vi "log analysis_gps.vi"() -> ()   [LabVIEW 2019] (continued)
37.37102056914,126.72168651879,7.9675,22.3000,0.3602,0.2584,-0.0273,-0.124586841,-0.381382122,33.473261992,0.4158,0.2973,0.5713,0.1134,0.0948,0.0862,0.2649,0.2392,5.1601,0f000001,0*eba26ee8\n\t", "INSPVAXA,USB3,0,50.5,FINESTEERING,2107,281412.850,02000000,471d,15824;INS_ALIGNMENT_COMPLETE,INS_RTKFIXED,37.37102404142,126.72168963423,7.9673,22.3000,0.3604,0.2695,-0.0148,-0.373966632,-0.606948860,33.415990980,0.4147,0.2955,0.5683,0.1128,0.0939,0.0847,0.2648,0.2392,5.1618,0f000001,0*2af052bc\n\t", "INSPVAXA,USB3,0,50.0,FINESTEERING,2107,281413.850,02000000,471d,15824;INS_ALIGNMENT_COMPLETE,INS_RTKFIXED,37.37102747823,126.72169275298,7.9678,22.3000,0.3771,0.2870,-0.0120,-0.268357218,-0.590747606,33.358928926,0.4139,0.2944,0.5647,0.1119,0.0930,0.0833,0.2648,0.2392,5.1630,0f000001,0*49d73869\n\t", "INSPVAXA,USB3,0,52.0,FINESTEERING,2107,281414.350,02000000,471d,15824;INS_ALIGNMENT_COMPLETE,INS_RTKFIXED,37.37102919906,126.72169428812,7.9675,22.3000,0.3604,0.2661,-0.0032,-0.659688126,-0.428969393,33.411905662,0.4132,0.2936,0.5618,0.1122,0.0937,0.0832,0.2648,0.2392,5.1641,0f000001,0*c98d060a\n\t", "INSPVAXA,USB3,0,44.5,FINESTEERING,2107,281415.350,02000000,471d,15824;INS_ALIGNMENT_COMPLETE,INS_RTKFIXED,37.37103267995,126.72169744869,7.9665,22.3000,0.3768,0.2993,-0.0116,-0.528478591,-0.759705931,33.438134045,0.4126,0.2929,0.5591,0.1118,0.0933,0.0820,0.2647,0.2392,5.1652,0f000001,0*581dc28c\n\t", "INSPVAXA,USB3,0,48.5,FINESTEERING,2107,281416.350,02000000,471d,15824;INS_ALIGNMENT_COMPLETE,INS_RTKFIXED,37.37103613052,126.72170062414,7.9635,22.3000,0.4087,0.2756,-0.0246,-0.725160800,-0.633419776,33.720037993,0.4128,0.2920,0.5564,0.1119,0.0930,0.0810,0.2647,0.2392,5.1665,0f000001,0*1631f0a5\n\t", "INSPVAXA,USB3,0,48.5,FINESTEERING,2107,281417.350,02000000,471d,15824;INS_ALIGNMENT_COMPLETE,INS_RTKFIXED,37.37103952444,126.72170377706,7.9632,22.3000,0.3570,0.2779,-0.0018,-0.570124026,-0.772949889,33.647986362,0.4118,0.2899,0.5509,0.1122,0.0932,0.0810,0.2645,0.2391,5.1675,0f000001,0*233b5573\n\t", "INSPVAXA,USB3,0,48.5,FINESTEERING,2107,281417.850,02000000,471d,15824;INS_ALIGNMENT_COMPLETE,INS_RTKFIXED,37.37104128675,126.72170534574,7.9659,22.3000,0.3708,0.2756,-0.0283,-0.789006262,-0.544112673,33.784716774,0.4118,0.2899,0.5509,0.1122,0.0932,0.0810,0.2645,0.2391,5.1675,0f000001,0*dc8c1e25\n\t", "INSPVAXA,USB3,0,49.0,FINESTEERING,2107,281418.850,02000000,471d,15824;INS_ALIGNMENT_COMPLETE,INS_RTKFIXED,37.37104464340,126.72170847296,7.9663,22.3000,0.3685,0.2500,0.0007,-0.664002073,-0.601650927,33.708955665,0.4113,0.2892,0.5478,0.1120,0.0929,0.0802,0.2644,0.2390,5.1688,0f000001,0*3627658d\n\t", "INSPVAXA,USB3,0,49.5,FINESTEERING,2107,281420.350,02000000,471d,15824;INS_ALIGNMENT_COMPLETE,INS_RTKFIXED,37.37104977182,126.72171326330,7.9681,22.3000,0.3654,0.2752,-0.0075,-0.486218413,-0.454617535,33.615388991,0.4147,0.2981,0.5609,0.1124,0.0945,0.0810,0.2643,0.2389,5.1711,0f000001,0*c1b15c55\n\t", "INSPVAXA,USB3,0,49.0,FINESTEERING,2107,281421.850,02000000,471d,15824;INS_ALIGNMENT_COMPLETE,INS_RTKFIXED,37.37105483304,126.72171804762,7.9714,22.3000,0.3720,0.2729,0.0059,-0.226869294,-0.357217167,33.322901739,0.4153,0.3006,0.5651,0.1122,0.0940,0.0806,0.2643,0.2388,5.1727,0f000001,0*c9d844c6\n\t", "INSPVAXA,USB3,0,50.0,FINESTEERING,2107,281440.400,02000000,471d,15824;INS_ALIGNMENT_COMPLETE,INS_RTKFIXED,37.37111948466,126.72177620543,7.8818,22.3000,0.3548,0.3148,0.0036,-0.259281902,-0.804731473,33.477876522,0.4069,0.2838,0.5238,0.1105,0.0914,0.0781,0.2627,0.2373,5.1917,0f000001,0*1022e28e\n\t", "INSPVAXA,USB3,0,47.0,FINESTEERING,2107,281451.400,02000000,471d,15824;INS_ALIGNMENT_COMPLETE,INS_RTKFIXED,37.37115737794,126.72181140198,7.8793,22.3000,0.3546,0.3544,0.0026,0.301499965,-0.418827265,36.616680382,0.4121,0.2951,0.5421,0.1113,0.0929,0.0791,0.2623,0.2370,5.2056,0f000001,0*452f9763\n\t", "INSPVAXA,USB3,0,44.5,FINESTEERING,2107,281452.400,02000000,471d,15824;INS_ALIGNMENT_COMPLETE,INS_RTKFIXED,37.37116058120,126.72181495507,7.8824,22.3000,0.3276,0.3265,-0.0468,0.306680390,-0.455879554,38.607757832,0.4139,0.2956,0.5455,0.1116,0.0928,0.0789,0.2623,0.2370,5.2072,0f000001,0*4613d5e8\n\t", "INSPVAXA,USB3,0,44.5,FINESTEERING,2107,281452.900,02000000,471d,15824;INS_ALIGNMENT_COMPLETE,INS_RTKFIXED,37.37116210966,126.72181674670,7.8822,22.3000,0.3215,0.3514,-0.0183,0.377751174,-0.234093113,39.308354629,0.4139,0.2956,0.5455,0.1116,0.0928,0.0789,0.2623,0.2370,5.2072,0f000001,0*f7d4e910\n\t", "INSPVAXA,USB3,0,49.0,FINESTEERING,2107,281453.400,02000000,471d,15824;INS_ALIGNMENT_COMPLETE,INS_RTKFIXED,37.37116361961,126.72181857489,7.8793,22.3000,0.3370,0.3634,-0.0294,0.431370913,-0.173130172,39.969478281,0.4147,0.2957,0.5475,0.1117,0.0928,0.0786,0.2622,0.2369,5.2083,0f000001,0*84da0b27\n\t", "INSPVAXA,USB3,0,49.0,FINESTEERING,2107,281453.900,02000000,471d,15824;INS_ALIGNMENT_COMPLETE,INS_RTKFIXED,37.37116508071,126.72182041170,7.8755,22.3000,0.3222,0.3708,0.0001,0.426257094,0.020843514,40.660737153,0.4147,0.2957,0.5475,0.1117,0.0928,0.0786,0.2622,0.2369,5.2083,0f000001,0*b9aa4650\n\t", "INSPVAXA,USB3,0,47.5,FINESTEERING,2107,281455.400,02000000,471d,15824;INS_ALIGNMENT_COMPLETE,INS_RTKFIXED,37.37116944200,126.72182606901,7.8692,22.3000,0.2987,0.3736,-0.0088,0.240749777,-0.612888046,41.923306200,0.4162,0.2974,0.5511,0.1132,0.0944,0.0792,0.2618,0.2366,5.2086,0f000001,0*c27b5d3d\n\t", "INSPVAXA,USB3,0,48.0,FINESTEERING,2107,281456.900,02000000,471d,15824;INS_ALIGNMENT_COMPLETE,INS_RTKFIXED,37.37117357948,126.72183178358,7.8608,22.3000,0.3100,0.3922,-0.0117,-0.041780079,0.015103018,42.742184550,0.4159,0.2958,0.5494,0.1140,0.0949,0.0793,0.2613,0.2363,5.2090,0f000001,0*a764cc08\n\t", "INSPVAXA,USB3,0,47.5,FINESTEERING,2107,281457.900,02008000,471d,15824;INS_ALIGNMENT_COMPLETE,INS_RTKFIXED,37.37117644696,126.72183567344,7.8614,22.3000,0.3036,0.3952,-0.0191,-0.435122492,0.297928497,42.865174724,0.4156,0.2944,0.5469,0.1149,0.0954,0.0797,0.2607,0.2357,5.2097,0f000001,0*67fee73b\n\t", "INSPVAXA,USB3,0,48.0,FINESTEERING,2107,281458.400,02008000,471d,15824;INS_ALIGNMENT_COMPLETE,INS_RTKFIXED,37.37117789762,126.72183765812,7.8605,22.3000,0.2663,0.3794,0.0055,-0.186627591,0.430628544,42.799150387,0.4156,0.2930,0.5449,0.1157,0.0959,0.0801,0.2599,0.2351,5.2111,0f000001,0*353aab58\n\t", "INSPVAXA,USB3,0,48.0,FINESTEERING,2107,281458.900,02008000,471d,15824;INS_ALIGNMENT_COMPLETE,INS_RTKFIXED,37.37117931784,126.72183956069,7.8626,22.3000,0.2674,0.3686,0.0176,-0.645699086,0.378450815,42.391957050,0.4156,0.2930,0.5449,0.1157,0.0959,0.0801,0.2599,0.2351,5.2111,0f000001,0*1d8f7f17\n\t", "INSPVAXA,USB3,0,50.5,FINESTEERING,2107,281459.900,02008000,471d,15824;INS_ALIGNMENT_COMPLETE,INS_RTKFIXED,37.37118223269,126.72184333763,7.8658,22.3000,0.2701,0.3610,0.0161,-0.453997018,0.223797272,40.778453294,0.4167,0.2944,0.5456,0.1164,0.0966,0.0809,0.2589,0.2343,5.2128,0f000001,0*32172057\n\t", "INSPVAXA,USB3,0,46.5,FINESTEERING,2107,281461.400,02008000,471d,15824;INS_ALIGNMENT_COMPLETE,INS_RTKFIXED,37.37118692248,126.72184864093,7.8697,22.3000,0.3068,0.3589,-0.0063,-0.709550175,-0.051664009,37.872013250,0.4180,0.2946,0.5458,0.1159,0.0960,0.0825,0.2566,0.2324,5.2151,0f000001,0*59364c44\n\t", "INSPVAXA,USB3,0,46.5,FINESTEERING,2107,281461.900,02008000,471d,15824;INS_ALIGNMENT_COMPLETE,INS_RTKFIXED,37.37118851997,126.72185034796,7.8716,22.3000,0.2953,0.3443,0.0004,-0.635296762,0.077766272,37.199284796,0.4180,0.2946,0.5458,0.1159,0.0960,0.0825,0.2566,0.2324,5.2151,0f000001,0*e7cf6597\n\t", "INSPVAXA,USB3,0,48.0,FINESTEERING,2107,281462.400,02008000,471d,15824;INS_ALIGNMENT_COMPLETE,INS_RTKFIXED,37.37119016469,126.72185198950,7.8718,22.3000,0.3140,0.3274,-0.0278,-0.753643784,0.303209826,36.783589938,0.4170,0.2921,0.5431,0.1150,0.0951,0.0832,0.2556,0.2316,5.2152,0f000001,0*71cc871c\n\t", "INSPVAXA,USB3,0,48.0,FINESTEERING,2107,281462.900,02008000,471d,15824;INS_ALIGNMENT_COMPLETE,INS_RTKFIXED,37.37119183431,126.72185366937,7.8730,22.3000,0.3211,0.3220,0.0114,-0.696465200,0.281664462,36.480823523,0.4170,0.2921,0.5431,0.1150,0.0951,0.0832,0.2556,0.2316,5.2152,0f000001,0*b2de4003\n\t", "INSPVAXA,USB3,0,48.5,FINESTEERING,2107,281463.400,02008000,471d,15824;INS_ALIGNMENT_COMPLETE,INS_RTKFIXED,37.37119351156,126.72185532212,7.8740,22.3000,0.2696,0.3105,-0.0010,-0.845084934,0.040994289,36.443862142,0.4171,0.2926,0.5444,0.1146,0.0951,0.0842,0.2547,0.2310,5.2149,0f000001,0*1ae650cc\n\t", "INSPVAXA,USB3,0,48.5,FINESTEERING,2107,281463.900,02008000,471d,15824;INS_ALIGNMENT_COMPLETE,INS_RTKFIXED,37.37119483302,126.72185668642,7.8760,22.3000,0.1153,0.1917,-0.0076,-0.816856486,-0.145545038,36.378444891,0.4171,0.2926,0.5444,0.1146,0.0951,0.0842,0.2547,0.2310,5.2149,0f000001,0*1c1cdd38\n\t", "INSPVAXA,USB3,0,45.5,FINESTEERING,2107,281464.400,02000000,471d,15824;INS_ALIGNMENT_COMPLETE,INS_RTKFIXED,37.37119579175,126.72185768591,7.8792,22.3000,0.1971,0.2398,0.0010,-0.742386203,-0.127943073,36.538622941,0.4195,0.2979,0.5527,0.1161,0.0973,0.0858,0.2541,0.2308,5.2143,0f000001,0*24dc1fe0\n\t", "INSPVAXA,USB3,0,45.5,FINESTEERING,2107,281464.900,02000000,471d,15824;INS_ALIGNMENT_COMPLETE,INS_RTKFIXED,37.37119672915,126.72185869204,7.8846,22.3000,0.1715,0.2230,-0.0041,-0.675547372,-0.136073790,36.631506264,0.4195,0.2979,0.5527,0.1161,0.0973,0.0858,0.2541,0.2308,5.2143,0f000001,0*e856a3ba\n\t", "INSPVAXA,USB3,0,49.0,FINESTEERING,2107,281465.400,02000000,471d,15824;INS_ALIGNMENT_COMPLETE,INS_RTKFIXED,37.37119777976,126.72185974580,7.8895,22.3000,0.1707,0.2152,-0.0021,-0.795130387,-0.134235456,36.862190913,0.4216,0.3036,0.5603,0.1136,0.0955,0.0851,0.2538,0.2307,5.2127,0f000001,0*3dceb74e\n\t", "INSPVAXA,USB3,0,49.0,FINESTEERING,2107,281465.900,02000000,471d,15824;INS_ALIGNMENT_COMPLETE,INS_RTKFIXED,37.37119882408,126.72186080871,7.8935,22.3000,0.1975,0.2377,-0.0103,-0.927101285,0.026313679,37.093891060,0.4216,0.3036,0.5603,0.1136,0.0955,0.0851,0.2538,0.2307,5.2127,0f000001,0*b32abc1e\n\t", "INSPVAXA,USB3,0,45.5,FINESTEERING,2107,281466.400,02000000,471d,15824;INS_ALIGNMENT_COMPLETE,INS_RTKFIXED,37.37119994764,126.72186191360,7.8953,22.3000,0.1896,0.2516,0.0024,-0.990040985,-0.050764765,37.290261699,0.4218,0.3053,0.5656,0.1126,0.0944,0.0842,0.2536,0.2306,5.2108,0f000001,0*ab7ec7da\n\t", "INSPVAXA,USB3,0,45.5,FINESTEERING,2107,281466.900,02000000,471d,15824;INS_ALIGNMENT_COMPLETE,INS_RTKFIXED,37.37120100149,126.72186298872,7.8973,22.3000,0.1935,0.2522,-0.0026,-0.854741520,-0.119099122,37.564308734,0.4218,0.3053,0.5656,0.1126,0.0944,0.0842,0.2536,0.2306,5.2108,0f000001,0*b7c581e3\n\t", "INSPVAXA,USB3,0,48.0,FINESTEERING,2107,281467.400,02000000,471d,15824;INS_ALIGNMENT_COMPLETE,INS_RTKFIXED,37.37120208153,126.72186408522,7.8997,22.3000,0.1778,0.2253,0.0049,-0.719912945,-0.270478243,38.035475922,0.4244,0.3113,0.5828,0.1121,0.0950,0.0843,0.2538,0.2306,5.2092,0f000001,0*8e9732d5\n\t", "INSPVAXA,USB3,0,48.0,FINESTEERING,2107,281467.900,02000000,471d,15824;INS_ALIGNMENT_COMPLETE,INS_RTKFIXED,37.37120312889,126.72186517178,7.9031,22.3000,0.2039,0.2426,0.0147,-0.720629061,-0.231870268,38.725653809,0.4244,0.3113,0.5828,0.1121,0.0950,0.0843,0.2538,0.2306,5.2092,0f000001,0*c758e7ce\n\t", "INSPVAXA,USB3,0,48.5,FINESTEERING,2107,281468.400,02000000,471d,15824;INS_ALIGNMENT_COMPLETE,INS_RTKFIXED,37.37120416086,126.72186625746,7.9066,22.3000,0.2025,0.2267,-0.0001,-0.736489084,-0.165649528,39.721937458,0.4260,0.3144,0.5975,0.1120,0.0953,0.0842,0.2539,0.2306,5.2089,0f000001,0*64b5bba4\n\t", "INSPVAXA,USB3,0,48.5,FINESTEERING,2107,281468.900,02000000,471d,15824;INS_ALIGNMENT_COMPLETE,INS_RTKFIXED,37.37120515414,126.72186733248,7.9096,22.3000,0.1860,0.2130,0.0062,-0.863833957,-0.176893088,40.861857992,0.4260,0.3144,0.5975,0.1120,0.0953,0.0842,0.2539,0.2306,5.2089,0f000001,0*48502021\n\t", "INSPVAXA,USB3,0,47.5,FINESTEERING,2107,281469.400,02000000,471d,15824;INS_ALIGNMENT_COMPLETE,INS_RTKFIXED,37.37120615783,126.72186845955,7.9127,22.3000,0.1833,0.2266,0.0157,-0.922756560,-0.128393101,41.953959499,0.4267,0.3157,0.6087,0.1119,0.0952,0.0838,0.2539,0.2306,5.2092,0f000001,0*9d6cc6cc\n\t", "INSPVAXA,USB3,0,47.5,FINESTEERING,2107,281469.900,02000000,471d,15824;INS_ALIGNMENT_COMPLETE,INS_RTKFIXED,37.37120711333,126.72186961218,7.9172,22.3000,0.1882,0.2386,0.0103,-0.812681162,-0.149481379,43.058831500,0.4267,0.3157,0.6087,0.1119,0.0952,0.0838,0.2539,0.2306,5.2092,0f000001,0*7e42c462\n\t", "INSPVAXA,USB3,0,48.0,FINESTEERING,2107,281470.400,02000000,471d,15824;INS_ALIGNMENT_COMPLETE,INS_RTKFIXED,37.37120802040,126.72187075599,7.9242,22.3000,0.1759,0.2315,0.0092,-0.712389099,-0.099720322,44.115258492,0.4228,0.3076,0.5975,0.1114,0.0938,0.0818,0.2538,0.2305,5.2102,0f000001,0*4e20fbfc\n\t", "INSPVAXA,USB3,0,48.0,FINESTEERING,2107,281470.900,02000000,471d,15824;INS_ALIGNMENT_COMPLETE,INS_RTKFIXED,37.37120891997,126.72187193685,7.9313,22.3000,0.1721,0.2325,0.0046,-0.682625247,-0.034958907,44.921832107,0.4228,0.3076,0.5975,0.1114,0.0938,0.0818,0.2538,0.2305,5.2102,0f000001,0*8a1ed08d\n\t", "INSPVAXA,USB3,0,44.5,FINESTEERING,2107,281471.400,02000000,471d,15824;INS_ALIGNMENT_COMPLETE,INS_RTKFIXED,37.37120978762,126.72187309291,7.9372,22.3000,0.1737,0.2402,0.0107,-0.896905071,0.182357572,45.734122702,0.4207,0.3039,0.5902,0.1115,0.0938,0.0806,0.2537,0.2305,5.2115,0f000001,0*f5531b04\n\t", "DUALANTENNAHEADINGA,USB3,0,44.5,FINESTEERING,2107,281471.900,02000000,d426,15824;SOL_COMPUTED,NARROW_FLOAT,-1.000000000,14.722629547,3.656694651,0.0,237.736404419,180.000000000,\"631T\",22,8,8,7,04,00,20,03*d908accb\n\t", "INSPVAXA,USB3,0,44.5,FINESTEERING,2107,281472.400,02000000,471d,15824;INS_ALIGNMENT_COMPLETE,INS_RTKFIXED,37.37121145223,126.72187546991,7.9481,22.3000,0.1558,0.2299,0.0072,-0.729574410,0.299435928,46.987178524,0.4186,0.2997,0.5808,0.1119,0.0940,0.0794,0.2536,0.2304,5.2130,0f000001,0*ceccfdc7\n\t", "DUALANTENNAHEADINGA,USB3,0,44.5,FINESTEERING,2107,281472.900,02000000,d426,15824;SOL_COMPUTED,NARROW_FLOAT,-1.000000000,19.887695313,3.310185432,0.0,262.944793701,180.000000000,\"631T\",19,8,8,7,04,00,20,03*e2f42a0a\n\t", "INSPVAXA,USB3,0,47.0,FINESTEERING,2107,281473.400,02000000,471d,15824;INS_ALIGNMENT_COMPLETE,INS_RTKFIXED,37.37121309194,126.72187787297,7.9563,22.3000,0.1608,0.2402,-0.0008,-0.731141510,0.324719411,47.702294704,0.4170,0.2975,0.5726,0.1126,0.0945,0.0786,0.2534,0.2303,5.2142,0f000001,0*03d357e2\n\t", "INSPVAXA,USB3,0,47.0,FINESTEERING,2107,281473.900,02000000,471d,15824;INS_ALIGNMENT_COMPLETE,INS_RTKFIXED,37.37121388735,126.72187905524,7.9593,22.3000,0.1511,0.2341,0.0050,-0.781655169,0.200652129,47.998434662,0.4170,0.2975,0.5726,0.1126,0.0945,0.0786,0.2534,0.2303,5.2142,0f000001,0*3307b87f\n\t", "INSPVAXA,USB3,0,50.0,FINESTEERING,2107,281474.400,02000000,471d,15824;INS_ALIGNMENT_COMPLETE,INS_RTKFIXED,37.37121466825,126.72188022113,7.9625,22.3000,0.1592,0.2409,0.0043,-0.925136185,0.519912466,48.197361455,0.4159,0.2959,0.5651,0.1133,0.0951,0.0780,0.2531,0.2301,5.2153,0f000001,0*acbf0539\n\t", "DUALANTENNAHEADINGA,USB3,0,50.0,FINESTEERING,2107,281474.900,02000000,d426,15824;SOL_COMPUTED,L1_FLOAT,-1.000000000,29.703872681,-19.285949707,0.0,227.925506592,180.000000000,\"631T\",19,7,7,7,04,00,20,02*438e8014\n\t", "INSPVAXA,USB3,0,48.0,FINESTEERING,2107,281475.400,02000000,471d,15824;INS_ALIGNMENT_COMPLETE,INS_RTKFIXED,37.37121622258,126.72188269700,7.9646,22.3000,0.1441,0.2253,0.0054,-0.653688748,0.578968322,48.454145381,0.4152,0.2943,0.5583,0.1140,0.0955,0.0776,0.2526,0.2297,5.2166,0f000001,0*7e585380\n\t", "INSPVAXA,USB3,0,48.0,FINESTEERING,2107,281475.900,02000000,471d,15824;INS_ALIGNMENT_COMPLETE,INS_RTKFIXED,37.37121692154,126.72188386600,7.9655,22.3000,0.1584,0.2123,0.0124,-0.619737810,0.551987551,48.617638369,0.4152,0.2943,0.5583,0.1140,0.0955,0.0776,0.2526,0.2297,5.2166,0f000001,0*cdba2d64\n\t", "INSPVAXA,USB3,0,46.5,FINESTEERING,2107,281476.400,02000000,471d,15824;INS_ALIGNMENT_COMPLETE,INS_RTKFIXED,37.37121768155,126.72188507525,7.9668,22.3000,0.1354,0.2014,0.0180,-0.822035432,0.378941407,48.791141972,0.4147,0.2931,0.5519,0.1146,0.0957,0.0772,0.2519,0.2292,5.2180,0f000001,0*1e1562b5\n\t", "INSPVAXA,USB3,0,46.5,FINESTEERING,2107,281476.900,02000000,471d,15824;INS_ALIGNMENT_COMPLETE,INS_RTKFIXED,37.37121850161,126.72188636358,7.9688,22.3000,0.1738,0.2367,0.0108,-1.201696541,-0.232647671,48.968391321,0.4147,0.2931,0.5519,0.1146,0.0957,0.0772,0.2519,0.2292,5.2180,0f000001,0*afd5e89e\n\t", "INSPVAXA,USB3,0,50.5,FINESTEERING,2107,281477.400,02000000,471d,15824;INS_ALIGNMENT_COMPLETE,INS_RTKFIXED,37.37121929078,126.72188763502,7.9707,22.3000,0.1401,0.2321,0.0104,-1.230903565,-0.339648847,49.051409136,0.4145,0.2921,0.5464,0.1152,0.0963,0.0770,0.2510,0.2285,5.2193,0f000001,0*fd6eca37\n\t", "DUALANTENNAHEADINGA,USB3,0,50.5,FINESTEERING,2107,281477.900,02000000,d426,15824;SOL_COMPUTED,NARROW_FLOAT,-1.000000000,24.973518372,-6.230041504,0.0,279.644378662,180.000000000,\"631T\",18,8,8,6,04,00,20,03*2ec7f676\n\t", "DUALANTENNAHEADINGA,USB3,0,45.5,FINESTEERING,2107,281478.400,02000000,d426,15824;SOL_COMPUTED,NARROW_FLOAT,-1.000000000,25.984382629,-14.421966553,0.0,321.839630127,180.000000000,\"631T\",19,7,7,6,04,00,20,03*c537a035\n\t", "INSPVAXA,USB3,0,45.5,FINESTEERING,2107,281478.900,02000000,471d,15824;INS_ALIGNMENT_COMPLETE,INS_RTKFIXED,37.37122160716,126.72189152509,7.9681,22.3000,0.1537,0.2575,-0.0106,-0.771104700,-0.770425381,49.241520291,0.4142,0.2902,0.5416,0.1154,0.0959,0.0768,0.2499,0.2277,5.2192,0f000001,0*21e6a269\n\t", "INSPVAXA,USB3,0,48.0,FINESTEERING,2107,281479.400,02000000,471d,15824;INS_ALIGNMENT_COMPLETE,INS_RTKFIXED,37.37122237259,126.72189283393,7.9651,22.3000,0.1293,0.2257,0.0059,-0.612587772,-1.097823401,49.383599810,0.4139,0.2890,0.5376,0.1159,0.0956,0.0767,0.2487,0.2267,5.2174,0f000001,0*f7632e7f\n\t", "INSPVAXA,USB3,0,48.0,FINESTEERING,2107,281479.900,02000000,471d,15824;INS_ALIGNMENT_COMPLETE,INS_RTKFIXED,37.37122311792,126.72189412346,7.9647,22.3000,0.1494,0.2660,0.0073,-0.587954124,-1.340332352,49.363469621,0.4139,0.2890,0.5376,0.1159,0.0956,0.0767,0.2487,0.2267,5.2174,0f000001,0*4724fb20\n\t", "DUALANTENNAHEADINGA,USB3,0,48.5,FINESTEERING,2107,281480.400,02000000,d426,15824;SOL_COMPUTED,L1_FLOAT,-1.000000000,38.387950897,-13.434600830,0.0,360.000000000,180.000000000,\"631T\",19,7,7,7,04,00,20,02*88d00c71\n\t", "DUALANTENNAHEADINGA,USB3,0,48.5,FINESTEERING,2107,281480.900,02000000,d426,15824;SOL_COMPUTED,L1_FLOAT,-1.000000000,37.718753815,-13.467346191,0.0,360.000000000,180.000000000,\"631T\",19,7,7,7,04,00,20,02*9128bd3b\n\t", "DUALANTENNAHEADINGA,USB3,0,46.5,FINESTEERING,2107,281481.400,02008000,d426,15824;SOL_COMPUTED,NARROW_FLOAT,-1.000000000,32.154727936,-10.026550293,0.0,255.698348999,180.000000000,\"631T\",21,8,8,7,04,00,20,03*90654ace\n\t", "INSPVAXA,USB3,0,46.5,FINESTEERING,2107,281481.900,02008000,471d,15824;INS_ALIGNMENT_COMPLETE,INS_RTKFIXED,37.37122611752,126.72189916270,7.9537,22.3000,0.1376,0.2362,0.0025,-0.095529965,-0.586716272,48.576302995,0.4131,0.2860,0.5308,0.1150,0.0939,0.0764,0.2461,0.2246,5.2038,0f000001,0*d4dc6a04\n\t", "INSPVAXA,USB3,0,43.0,FINESTEERING,2107,281482.400,02008000,471d,15824;INS_ALIGNMENT_COMPLETE,INS_RTKFIXED,37.37122693129,126.72190044241,7.9507,22.3000,0.1400,0.2344,0.0009,-0.286718935,-0.542573010,48.417760410,0.4129,0.2856,0.5284,0.1143,0.0930,0.0764,0.2448,0.2237,5.1963,0f000001,0*4b0c873a\n\t", "DUALANTENNAHEADINGA,USB3,0,43.0,FINESTEERING,2107,281482.900,02008000,d426,15824;SOL_COMPUTED,NARROW_FLOAT,-1.000000000,25.759243011,-24.488281250,0.0,296.027648926,180.000000000,\"631T\",21,7,7,7,04,00,20,03*7949ae50\n\t", "DUALANTENNAHEADINGA,USB3,0,49.0,FINESTEERING,2107,281483.400,02008000,d426,15824;SOL_COMPUTED,NARROW_FLOAT,-1.000000000,21.557176590,-28.431182861,0.0,309.766693115,180.000000000,\"631T\",20,8,8,7,04,00,20,03*24e13096\n\t", "INSPVAXA,USB3,0,49.0,FINESTEERING,2107,281483.900,02008000,471d,15824;INS_ALIGNMENT_COMPLETE,INS_RTKFIXED,37.37122933882,126.72190424641,7.9440,22.3000,0.1298,0.2079,0.0016,-0.555050997,-0.344115137,48.037628133,0.4121,0.2847,0.5256,0.1130,0.0922,0.0763,0.2437,0.2229,5.1908,0f000001,0*4fcd94af\n\t", "DUALANTENNAHEADINGA,USB3,0,50.0,FINESTEERING,2107,281484.400,02008000,d426,15824;SOL_COMPUTED,L1_FLOAT,-1.000000000,37.365016937,-21.970794678,0.0,360.000000000,180.000000000,\"631T\",19,7,7,7,04,00,20,02*e133e505\n\t", "INSPVAXA,USB3,0,50.0,FINESTEERING,2107,281484.900,02008000,471d,15824;INS_ALIGNMENT_COMPLETE,INS_RTKFIXED,37.37123096597,126.72190680248,7.9384,22.3000,0.1511,0.2333,-0.0078,-0.410489938,-0.523354884,48.112153719,0.4115,0.2844,0.5237,0.1121,0.0916,0.0762,0.2426,0.2223,5.1884,0f000001,0*a1f40ef1\n\t", "DUALANTENNAHEADINGA,USB3,0,47.5,FINESTEERING,2107,281485.400,02000000,d426,15824;SOL_COMPUTED,NARROW_FLOAT,-1.000000000,34.474456787,-26.341827393,0.0,271.964752197,180.000000000,\"631T\",20,7,7,7,04,00,20,03*cc121194\n\t", "INSPVAXA,USB3,0,47.5,FINESTEERING,2107,281485.900,02000000,471d,15824;INS_ALIGNMENT_COMPLETE,INS_RTKFIXED,37.37123256957,126.72190927922,7.9317,22.3000,0.1299,0.2173,-0.0089,-0.426845608,-0.944074849,48.432879849,0.4110,0.2838,0.5218,0.1115,0.0911,0.0761,0.2417,0.2218,5.1881,0f000001,0*ee8ace9e\n\t", "DUALANTENNAHEADINGA,USB3,0,48.0,FINESTEERING,2107,281486.400,02000000,d426,15824;SOL_COMPUTED,L1_FLOAT,-1.000000000,34.864692688,-21.694915771,0.0,360.000000000,180.000000000,\"631T\",20,7,7,7,04,00,20,02*de044530\n\t", "DUALANTENNAHEADINGA,USB3,0,48.0,FINESTEERING,2107,281486.900,02000000,d426,15824;SOL_COMPUTED,L1_FLOAT,-1.000000000,35.417118073,-21.326538086,0.0,360.000000000,180.000000000,\"631T\",20,7,7,7,04,00,20,02*a4d3627b\n\t", "INSPVAXA,USB3,0,48.5,FINESTEERING,2107,281487.400,02000000,471d,15824;INS_ALIGNMENT_COMPLETE,INS_RTKFIXED,37.37123510484,126.72191313192,7.9239,22.3000,0.1508,0.2267,-0.0041,-0.710611469,-0.697297129,49.092383754,0.4097,0.2833,0.5200,0.1105,0.0907,0.0760,0.2404,0.2213,5.1897,0f000001,0*65fc2fbf\n\t", "INSPVAXA,USB3,0,48.5,FINESTEERING,2107,281487.900,02000000,471d,15824;INS_ALIGNMENT_COMPLETE,INS_RTKFIXED,37.37123588578,126.72191437981,7.9197,22.3000,0.1455,0.2377,-0.0129,-0.683157100,-0.548580830,49.602033608,0.4097,0.2833,0.5200,0.1105,0.0907,0.0760,0.2404,0.2213,5.1897,0f000001,0*fc400f11\n\t", "INSPVAXA,USB3,0,47.5,FINESTEERING,2107,281488.400,02000000,471d,15824;INS_ALIGNMENT_COMPLETE,INS_RTKFIXED,37.37123668548,126.72191567046,7.9173,22.3000,0.1286,0.2563,0.0010,-0.700638856,-0.301855154,50.490709534,0.4091,0.2828,0.5195,0.1103,0.0906,0.0760,0.2400,0.2212,5.1909,0f000001,0*20940426\n\t", "INSPVAXA,USB3,0,47.5,FINESTEERING,2107,281488.900,02000000,471d,15824;INS_ALIGNMENT_COMPLETE,INS_RTKFIXED,37.37123745255,126.72191698522,7.9152,22.3000,0.1363,0.2513,-0.0110,-0.588840465,-0.298661481,51.824057860,0.4091,0.2828,0.5195,0.1103,0.0906,0.0760,0.2400,0.2212,5.1909,0f000001,0*3253a0a6\n\t", "DUALANTENNAHEADINGA,USB3,0,48.5,FINESTEERING,2107,281489.400,02000000,d426,15824;SOL_COMPUTED,NARROW_FLOAT,-1.000000000,34.332912445,-16.076080322,0.0,273.294891357,180.000000000,\"631T\",21,7,7,7,04,00,20,02*2e8f18b8\n\t", "DUALANTENNAHEADINGA,USB3,0,48.5,FINESTEERING,2107,281489.900,02000000,d426,15824;SOL_COMPUTED,NARROW_FLOAT,-1.000000000,35.701751709,-15.985229492,0.0,272.194824219,180.000000000,\"631T\",19,7,7,7,04,00,20,03*54912f65\n\t", "DUALANTENNAHEADINGA,USB3,0,49.0,FINESTEERING,2107,281490.400,02000000,d426,15824;SOL_COMPUTED,L1_FLOAT,-1.000000000,33.157665253,-11.030181885,0.0,245.857955933,180.000000000,\"631T\",19,7,7,7,04,00,20,02*0068c7a6\n\t", "INSPVAXA,USB3,0,49.0,FINESTEERING,2107,281490.900,02000000,471d,15824;INS_ALIGNMENT_COMPLETE,INS_RTKFIXED,37.37124025850,126.72192244807,7.9063,22.3000,0.0958,0.2597,0.0085,-0.741191829,-0.240876601,58.109405467,0.4082,0.2817,0.5177,0.1106,0.0906,0.0758,0.2393,0.2210,5.1939,0f000001,0*b3d0469a\n\t", "INSPVAXA,USB3,0,49.0,FINESTEERING,2107,281491.400,02000000,471d,15824;INS_ALIGNMENT_COMPLETE,INS_RTKFIXED,37.37124087093,126.72192387521,7.9056,22.3000,0.0957,0.2456,-0.0018,-0.666118734,-0.163871029,59.496681270,0.4086,0.2815,0.5172,0.1112,0.0911,0.0758,0.2390,0.2209,5.1955,0f000001,0*877ace1f\n\t", "DUALANTENNAHEADINGA,USB3,0,49.0,FINESTEERING,2107,281491.900,02000000,d426,15824;SOL_COMPUTED,L1_FLOAT,-1.000000000,38.072498322,-12.872985840,0.0,241.422912598,180.000000000,\"631T\",19,9,9,9,04,00,20,22*0432346e\n\t", "DUALANTENNAHEADINGA,USB3,0,48.5,FINESTEERING,2107,281492.400,02000000,d426,15824;SOL_COMPUTED,L1_FLOAT,-1.000000000,43.679172516,-11.013610840,0.0,278.657897949,180.000000000,\"631T\",19,9,9,9,04,00,20,22*bdfbef21\n\t", "DUALANTENNAHEADINGA,USB3,0,48.5,FINESTEERING,2107,281492.900,02000000,d426,15824;SOL_COMPUTED,L1_FLOAT,-1.000000000,44.166721344,-11.721832275,0.0,281.896148682,180.000000000,\"631T\",20,9,9,9,04,00,20,22*48a6c000\n\t", "INSPVAXA,USB3,0,42.5,FINESTEERING,2107,281493.400,02000000,471d,15824;INS_ALIGNMENT_COMPLETE,INS_RTKFIXED,37.37124296430,126.72192966667,7.9049,22.3000,0.0753,0.2701,-0.0078,-0.323936505,-0.201612973,63.426537614,0.4097,0.2821,0.5162,0.1137,0.0933,0.0757,0.2379,0.2204,5.1978,0f000001,0*1142f323\n\t", "INSPVAXA,USB3,0,42.5,FINESTEERING,2107,281493.900,02000000,471d,15824;INS_ALIGNMENT_COMPLETE,INS_RTKFIXED,37.37124340358,126.72193109595,7.9039,22.3000,0.0669,0.2621,-0.0103,-0.274820593,-0.183280206,64.003294915,0.4097,0.2821,0.5162,0.1137,0.0933,0.0757,0.2379,0.2204,5.1978,0f000001,0*917919f7\n\t", "DUALANTENNAHEADINGA,USB3,0,47.0,FINESTEERING,2107,281494.400,02000000,d426,15824;SOL_COMPUTED,L1_FLOAT,-1.000000000,39.924659729,-8.854888916,0.0,360.000000000,180.000000000,\"631T\",19,7,7,7,04,00,20,02*f82ff11c\n\t", "DUALANTENNAHEADINGA,USB3,0,47.0,FINESTEERING,2107,281494.900,02000000,d426,15824;SOL_COMPUTED,L1_FLOAT,-1.000000000,40.630737305,-7.196624756,0.0,360.000000000,180.000000000,\"631T\",19,7,7,7,04,00,20,02*f7322ed7\n\t", "DUALANTENNAHEADINGA,USB3,0,52.0,FINESTEERING,2107,281495.400,02000000,d426,15824;SOL_COMPUTED,L1_FLOAT,-1.000000000,40.645214081,-8.830108643,0.0,360.000000000,180.000000000,\"631T\",18,7,7,7,04,00,20,02*8609447b\n\t", "INSPVAXA,USB3,0,52.0,FINESTEERING,2107,281495.900,02000000,471d,15824;INS_ALIGNMENT_COMPLETE,INS_RTKFIXED,37.37124512541,126.72193695200,7.9047,22.3000,0.0463,0.2469,-0.0072,0.000083390,-0.348047959,65.534193450,0.4125,0.2835,0.5158,0.1165,0.0957,0.0756,0.2356,0.2190,5.1978,0f000001,0*14e6bfac\n\t", "DUALANTENNAHEADINGA,USB3,0,49.0,FINESTEERING,2107,281496.400,02000000,d426,15824;SOL_COMPUTED,NARROW_FLOAT,-1.000000000,36.124023438,-7.202545166,0.0,327.448486328,180.000000000,\"631T\",21,7,7,7,04,00,20,03*2df9ffe6\n\t", "DUALANTENNAHEADINGA,USB3,0,49.0,FINESTEERING,2107,281496.900,02000000,d426,15824;SOL_COMPUTED,NARROW_FLOAT,-1.000000000,36.800415039,-8.357086182,0.0,335.148284912,180.000000000,\"631T\",21,7,7,7,04,00,20,03*89694ba0\n\t", "DUALANTENNAHEADINGA,USB3,0,45.5,FINESTEERING,2107,281497.400,02000000,d426,15824;SOL_COMPUTED,NARROW_FLOAT,-1.000000000,35.379425049,-14.173278809,0.0,252.907455444,180.000000000,\"631T\",20,8,8,7,04,00,20,03*7b0cb3e2\n\t", "DUALANTENNAHEADINGA,USB3,0,45.5,FINESTEERING,2107,281497.900,02000000,d426,15824;SOL_COMPUTED,NARROW_FLOAT,-1.000000000,35.681621552,-15.419891357,0.0,255.079315186,180.000000000,\"631T\",18,8,8,7,04,00,20,03*3e48e9bf\n\t", "DUALANTENNAHEADINGA,USB3,0,47.0,FINESTEERING,2107,281498.400,02008000,d426,15824;SOL_COMPUTED,L1_FLOAT,-1.000000000,40.500751495,-12.284759521,0.0,360.000000000,180.000000000,\"631T\",19,7,7,7,04,00,20,02*8d7c2d6f\n\t", "DUALANTENNAHEADINGA,USB3,0,46.5,FINESTEERING,2107,281499.400,02008000,d426,15824;SOL_COMPUTED,L1_FLOAT,-1.000000000,47.084907532,-15.694274902,0.0,360.000000000,180.000000000,\"631T\",19,7,7,7,04,00,20,02*f0de5a60\n\t", "DUALANTENNAHEADINGA,USB3,0,46.5,FINESTEERING,2107,281499.900,02008000,d426,15824;SOL_COMPUTED,L1_FLOAT,-1.000000000,46.870197296,-16.724273682,0.0,360.000000000,180.000000000,\"631T\",18,7,7,7,04,00,20,02*32f34491\n\t", "DUALANTENNAHEADINGA,USB3,0,48.5,FINESTEERING,2107,281500.400,02008000,d426,15824;SOL_COMPUTED,L1_FLOAT,-1.000000000,46.407375336,-16.426940918,0.0,360.000000000,180.000000000,\"631T\",18,7,7,7,04,00,20,02*243e6382\n\t", "DUALANTENNAHEADINGA,USB3,0,48.5,FINESTEERING,2107,281500.900,02008000,d426,15824;SOL_COMPUTED,L1_FLOAT,-1.000000000,46.192268372,-15.498413086,0.0,360.000000000,180.000000000,\"631T\",17,7,7,7,04,00,20,02*d63e23bb\n\t", "DUALANTENNAHEADINGA,USB3,0,48.5,FINESTEERING,2107,281501.400,02008000,d426,15824;SOL_COMPUTED,L1_FLOAT,-1.000000000,48.142848969,-21.188415527,0.0,360.000000000,180.000000000,\"631T\",17,7,7,7,04,00,20,02*7f9c1701\n\t", "DUALANTENNAHEADINGA,USB3,0,48.5,FINESTEERING,2107,281501.900,02008000,d426,15824;SOL_COMPUTED,L1_FLOAT,-1.000000000,48.243919373,-21.323577881,0.0,360.000000000,180.000000000,\"631T\",18,7,7,7,04,00,20,02*9b797559\n\t", "DUALANTENNAHEADINGA,USB3,0,51.0,FINESTEERING,2107,281502.400,02000000,d426,15824;SOL_COMPUTED,L1_FLOAT,-1.000000000,54.417652130,-31.199645996,0.0,360.000000000,180.000000000,\"631T\",17,7,7,7,04,00,20,02*139cf8a7\n\t", "DUALANTENNAHEADINGA,USB3,0,51.0,FINESTEERING,2107,281504.900,02000000,d426,15824;SOL_COMPUTED,NARROW_FLOAT,-1.000000000,45.458030701,-24.170471191,0.0,349.614562988,180.000000000,\"631T\",18,7,7,7,04,00,20,03*3763f111\n\t", "DUALANTENNAHEADINGA,USB3,0,47.0,FINESTEERING,2107,281506.400,02000000,d426,15824;SOL_COMPUTED,L1_FLOAT,-1.000000000,47.490772247,-15.120605469,0.0,360.000000000,180.000000000,\"631T\",20,7,7,7,04,00,20,02*6c842724\n\t", "DUALANTENNAHEADINGA,USB3,0,47.0,FINESTEERING,2107,281506.900,02000000,d426,15824;SOL_COMPUTED,L1_FLOAT,-1.000000000,47.711154938,-15.635345459,0.0,360.000000000,180.000000000,\"631T\",18,7,7,7,04,00,20,02*a44c5d4d\n\t", "DUALANTENNAHEADINGA,USB3,0,47.5,FINESTEERING,2107,281507.400,02000000,d426,15824;SOL_COMPUTED,NARROW_FLOAT,-1.000000000,42.099899292,-18.667358398,0.0,341.481109619,180.000000000,\"631T\",17,7,7,7,04,00,20,03*b5db1bef\n\t", "INSPVAXA,USB3,0,47.5,FINESTEERING,2107,281507.950,02000000,471d,15824;INS_ALIGNMENT_COMPLETE,INS_RTKFIXED,37.37125380804,126.72197426812,7.8769,22.3000,-0.0203,0.2606,-0.0150,0.201245645,-0.677592145,78.627863448,0.4158,0.2828,0.5148,0.1162,0.0939,0.0753,0.2087,0.2003,5.2095,0f000001,0*4e226b57\n\t", "DUALANTENNAHEADINGA,USB3,0,49.0,FINESTEERING,2107,281508.900,02000000,d426,15824;SOL_COMPUTED,L1_FLOAT,-1.000000000,44.870548248,-15.658569336,0.0,360.000000000,180.000000000,\"631T\",16,7,7,7,04,00,20,02*b0c8f4ea\n\t", "DUALANTENNAHEADINGA,USB3,0,48.0,FINESTEERING,2107,281509.400,02000000,d426,15824;SOL_COMPUTED,NARROW_FLOAT,-1.000000000,43.414321899,-11.001037598,0.0,331.000732422,180.000000000,\"631T\",16,7,7,7,04,00,20,03*47deaf74\n\t", "INSPVAXA,USB3,0,48.0,FINESTEERING,2107,281509.950,02000000,471d,15824;INS_ALIGNMENT_COMPLETE,INS_RTKFIXED,37.37125445097,126.72198074425,7.8673,22.3000,-0.0085,0.2660,-0.0026,-0.121772207,-0.607137029,81.065804036,0.4154,0.2822,0.5141,0.1167,0.0945,0.0753,0.2051,0.1982,5.2122,0f000001,0*3f1eba48\n\t", "INSPVAXA,USB3,0,49.0,FINESTEERING,2107,281510.950,02000000,471d,15824;INS_ALIGNMENT_COMPLETE,INS_RTKFIXED,37.37125469386,126.72198394017,7.8637,22.3000,-0.0196,0.2391,0.0072,0.076200497,-0.660108168,81.872681824,0.4156,0.2817,0.5136,0.1168,0.0948,0.0753,0.2032,0.1971,5.2137,0f000001,0*0481949b\n\t", "DUALANTENNAHEADINGA,USB3,0,46.5,FINESTEERING,2107,281511.400,02000000,d426,15824;SOL_COMPUTED,L1_FLOAT,-1.000000000,48.665706635,-11.851898193,0.0,360.000000000,180.000000000,\"631T\",23,7,7,7,04,00,20,02*002e390f\n\t", "DUALANTENNAHEADINGA,USB3,0,46.5,FINESTEERING,2107,281511.900,02000000,d426,15824;SOL_COMPUTED,L1_FLOAT,-1.000000000,49.675540924,-13.921539307,0.0,360.000000000,180.000000000,\"631T\",22,7,7,7,04,00,20,02*d8f1bbd6\n\t", "DUALANTENNAHEADINGA,USB3,0,49.5,FINESTEERING,2107,281513.900,02000000,d426,15824;SOL_COMPUTED,NARROW_FLOAT,-1.000000000,44.284626007,-19.218811035,0.0,360.000000000,180.000000000,\"631T\",20,7,7,7,04,00,20,02*521f05df\n\t", "INSPVAXA,USB3,0,49.5,FINESTEERING,2107,281514.450,02000000,471d,15824;INS_ALIGNMENT_COMPLETE,INS_RTKFIXED,37.37125536287,126.72199528915,7.8355,22.3000,-0.0378,0.2111,0.0002,0.439353966,-1.869293948,83.706823159,0.4159,0.2810,0.5124,0.1164,0.0945,0.0753,0.1954,0.1923,5.2170,0f000001,0*665bd911\n\t", "DUALANTENNAHEADINGA,USB3,0,49.0,FINESTEERING,2107,281515.400,02000000,d426,15824;SOL_COMPUTED,L1_FLOAT,-1.000000000,38.143417358,-18.359069824,0.0,274.915802002,180.000000000,\"631T\",19,9,9,9,04,00,20,22*781bfffa\n\t", "INSPVAXA,USB3,0,49.0,FINESTEERING,2107,281515.950,02000000,471d,15824;INS_ALIGNMENT_COMPLETE,INS_RTKFIXED,37.37125550223,126.72200026219,7.8204,22.3000,-0.0297,0.2447,-0.0075,0.993050035,-2.146972664,84.455014366,0.4154,0.2808,0.5121,0.1158,0.0940,0.0753,0.1936,0.1911,5.2166,0f000001,0*f4a4a55a\n\t", "INSPVAXA,USB3,0,49.5,FINESTEERING,2107,281516.950,02000000,471d,15824;INS_ALIGNMENT_COMPLETE,INS_RTKFIXED,37.37125561676,126.72200346260,7.8093,22.3000,-0.0298,0.2388,-0.0036,0.877000312,-2.356206716,84.738207188,0.4150,0.2807,0.5119,0.1151,0.0935,0.0753,0.1918,0.1900,5.2169,0f000001,0*302168dd\n\t", "INSPVAXA,USB3,0,49.0,FINESTEERING,2107,281517.950,02000000,471d,15824;INS_ALIGNMENT_COMPLETE,INS_RTKFIXED,37.37125568444,126.72200682151,7.7945,22.3000,-0.0192,0.2217,-0.0192,1.425946451,-2.539207007,85.090836671,0.4150,0.2807,0.5120,0.1146,0.0931,0.0754,0.1902,0.1890,5.2177,0f000001,0*9a7264e1\n\t", "DUALANTENNAHEADINGA,USB3,0,47.0,FINESTEERING,2107,281518.400,02000000,d426,15824;SOL_COMPUTED,L1_FLOAT,-1.000000000,42.740367889,-32.075164795,0.0,319.860687256,180.000000000,\"631T\",19,9,9,9,04,00,20,22*d53a90ac\n\t", "INSPVAXA,USB3,0,47.0,FINESTEERING,2107,281518.950,02000000,471d,15824;INS_ALIGNMENT_COMPLETE,INS_RTKFIXED,37.37125573981,126.72201005340,7.7819,22.3000,-0.0255,0.2627,-0.0105,1.331964681,-2.358060852,85.490717042,0.4145,0.2807,0.5123,0.1139,0.0926,0.0754,0.1888,0.1882,5.2187,0f000001,0*a7b8d42f\n\t", "DUALANTENNAHEADINGA,USB3,0,48.5,FINESTEERING,2107,281519.900,02000000,d426,15824;SOL_COMPUTED,L1_FLOAT,-1.000000000,50.327861786,-37.477569580,0.0,318.157135010,180.000000000,\"631T\",19,6,6,6,04,00,20,02*633b419f\n\t", "INSPVAXA,USB3,0,50.5,FINESTEERING,2107,281520.450,02000000,471d,15824;INS_ALIGNMENT_COMPLETE,INS_RTKFIXED,37.37125585823,126.72201493380,7.7618,22.3000,-0.0241,0.3156,-0.0229,0.726950226,-1.736335122,85.946194280,0.4135,0.2799,0.5121,0.1130,0.0919,0.0756,0.1864,0.1868,5.2210,0f000001,0*82c9f176\n\t", "INSPVAXA,USB3,0,50.5,FINESTEERING,2107,281520.950,02000000,471d,15824;INS_ALIGNMENT_COMPLETE,INS_RTKFIXED,37.37125587974,126.72201671987,7.7507,22.3000,-0.0399,0.2427,-0.0046,0.656221205,-1.866737279,86.202077970,0.4135,0.2799,0.5121,0.1130,0.0919,0.0756,0.1864,0.1868,5.2210,0f000001,0*df1ef1f5\n\t", "INSPVAXA,USB3,0,46.5,FINESTEERING,2107,281521.950,02000000,471d,15824;INS_ALIGNMENT_COMPLETE,INS_RTKFIXED,37.37125587376,126.72201976127,7.7406,22.3000,-0.0074,0.2755,0.0027,0.545815584,-0.620038116,86.574318389,0.4139,0.2794,0.5123,0.1122,0.0918,0.0756,0.1854,0.1863,5.2222,0f000001,0*d388b8b0\n\t", "INSPVAXA,USB3,0,50.0,FINESTEERING,2107,281522.450,02000000,471d,15824;INS_ALIGNMENT_COMPLETE,INS_RTKFIXED,37.37125594460,126.72202128419,7.7372,22.3000,-0.0117,0.2731,-0.0129,-0.654259534,-0.666330623,86.875849096,0.4136,0.2787,0.5123,0.1124,0.0922,0.0756,0.1845,0.1859,5.2224,0f000001,0*d87bbb5d\n\t", "INSPVAXA,USB3,0,50.0,FINESTEERING,2107,281522.950,02000000,471d,15824;INS_ALIGNMENT_COMPLETE,INS_RTKFIXED,37.37125596414,126.72202295836,7.7342,22.3000,-0.0333,0.2828,-0.0046,-1.065587948,-0.382081597,87.029767697,0.4136,0.2787,0.5123,0.1124,0.0922,0.0756,0.1845,0.1859,5.2224,0f000001,0*2edab05f\n\t", "INSPVAXA,USB3,0,50.0,FINESTEERING,2107,281523.450,02000000,471d,15824;INS_ALIGNMENT_COMPLETE,INS_RTKFIXED,37.37125596415,126.72202454079,7.7319,22.3000,-0.0484,0.2411,-0.0123,-1.089747503,0.421440588,87.147048457,0.4141,0.2781,0.5123,0.1124,0.0923,0.0755,0.1837,0.1856,5.2192,0f000001,0*53e95b2b\n\t", "INSPVAXA,USB3,0,50.0,FINESTEERING,2107,281523.950,02000000,471d,15824;INS_ALIGNMENT_COMPLETE,INS_RTKFIXED,37.37125592914,126.72202612283,7.7345,22.3000,-0.0454,0.2984,-0.0075,-0.788968159,0.571056615,87.325442989,0.4141,0.2781,0.5123,0.1124,0.0923,0.0755,0.1837,0.1856,5.2192,0f000001,0*39ccc3b7\n\t", "INSPVAXA,USB3,0,50.0,FINESTEERING,2107,281524.450,02000000,471d,15824;INS_ALIGNMENT_COMPLETE,INS_RTKFIXED,37.37125593181,126.72202769254,7.7370,22.3000,-0.0382,0.2867,-0.0035,-1.197739356,0.920892759,87.655051313,0.4147,0.2775,0.5122,0.1123,0.0915,0.0754,0.1830,0.1854,5.2111,0f000001,0*f9d72c69\n\t", "INSPVAXA,USB3,0,50.0,FINESTEERING,2107,281524.950,02000000,471d,15824;INS_ALIGNMENT_COMPLETE,INS_RTKFIXED,37.37125591109,126.72202930356,7.7399,22.3000,-0.0391,0.2791,0.0008,-1.548464832,1.177525409,87.896240869,0.4147,0.2775,0.5122,0.1123,0.0915,0.0754,0.1830,0.1854,5.2111,0f000001,0*83d571d9\n\t", "INSPVAXA,USB3,0,48.5,FINESTEERING,2107,281526.450,02000000,471d,15824;INS_ALIGNMENT_COMPLETE,INS_RTKFIXED,37.37125584524,126.72203425117,7.7504,22.3000,-0.0601,0.2713,0.0036,-1.381885120,0.929156206,88.315257538,0.4157,0.2770,0.5121,0.1113,0.0909,0.0752,0.1819,0.1851,5.1872,0f000001,0*291f5036\n\t", "INSPVAXA,USB3,0,48.5,FINESTEERING,2107,281526.950,02000000,471d,15824;INS_ALIGNMENT_COMPLETE,INS_RTKFIXED,37.37125579589,126.72203592362,7.7537,22.3000,-0.0480,0.2913,0.0058,-1.173614643,0.491373435,88.468098550,0.4157,0.2770,0.5121,0.1113,0.0909,0.0752,0.1819,0.1851,5.1872,0f000001,0*d2925fbc\n\t", "INSPVAXA,USB3,0,48.0,FINESTEERING,2107,281527.950,02000000,471d,15824;INS_ALIGNMENT_COMPLETE,INS_RTKFIXED,37.37125572987,126.72203920387,7.7658,22.3000,-0.0524,0.2827,0.0097,-1.037615200,0.271270878,88.658127603,0.4153,0.2771,0.5121,0.1104,0.0905,0.0752,0.1816,0.1850,5.1752,0f000001,0*cc65e324\n\t", "INSPVAXA,USB3,0,50.0,FINESTEERING,2107,281528.450,02000000,471d,15824;INS_ALIGNMENT_COMPLETE,INS_RTKFIXED,37.37125569644,126.72204084208,7.7707,22.3000,-0.0559,0.2951,0.0043,-0.934405455,0.587306829,88.715451510,0.4138,0.2768,0.5118,0.1101,0.0902,0.0751,0.1812,0.1850,5.1681,0f000001,0*38aa8fdd\n\t", "INSPVAXA,USB3,0,50.0,FINESTEERING,2107,281528.950,02000000,471d,15824;INS_ALIGNMENT_COMPLETE,INS_RTKFIXED,37.37125565087,126.72204247728,7.7739,22.3000,-0.0479,0.2916,0.0001,-0.888338031,0.781445457,88.804413207,0.4138,0.2768,0.5118,0.1101,0.0902,0.0751,0.1812,0.1850,5.1681,0f000001,0*a995e794\n\t", "INSPVAXA,USB3,0,45.5,FINESTEERING,2107,281529.450,02000000,471d,15824;INS_ALIGNMENT_COMPLETE,INS_RTKFIXED,37.37125561815,126.72204405961,7.7805,22.3000,-0.0427,0.2707,0.0059,-0.985512427,0.998310951,88.869085357,0.4125,0.2769,0.5116,0.1099,0.0902,0.0751,0.1810,0.1850,5.1659,0f000001,0*0269fb35\n\t", "INSPVAXA,USB3,0,45.5,FINESTEERING,2107,281529.950,02000000,471d,15824;INS_ALIGNMENT_COMPLETE,INS_RTKFIXED,37.37125556208,126.72204568853,7.7886,22.3000,-0.0448,0.2875,0.0039,-0.937316119,0.971606302,88.876668498,0.4125,0.2769,0.5116,0.1099,0.0902,0.0751,0.1810,0.1850,5.1659,0f000001,0*914c1aec\n\t", "INSPVAXA,USB3,0,49.0,FINESTEERING,2107,281530.450,02000000,471d,15824;INS_ALIGNMENT_COMPLETE,INS_RTKFIXED,37.37125551286,126.72204733678,7.7958,22.3000,-0.0391,0.2940,0.0024,-0.847859787,0.758698314,88.842002918,0.4116,0.2768,0.5112,0.1098,0.0901,0.0751,0.1808,0.1849,5.1659,0f000001,0*a7731e83\n\t", "INSPVAXA,USB3,0,49.0,FINESTEERING,2107,281530.950,02000000,471d,15824;INS_ALIGNMENT_COMPLETE,INS_RTKFIXED,37.37125545025,126.72204900061,7.8022,22.3000,-0.0360,0.2787,-0.0016,-0.812645512,0.794768831,88.914177046,0.4116,0.2768,0.5112,0.1098,0.0901,0.0751,0.1808,0.1849,5.1659,0f000001,0*55377a3b\n\t", "INSPVAXA,USB3,0,48.5,FINESTEERING,2107,281531.450,02000000,471d,15824;INS_ALIGNMENT_COMPLETE,INS_RTKFIXED,37.37125540137,126.72205063289,7.8075,22.3000,-0.0425,0.2797,0.0032,-0.889554517,0.869596367,88.992176965,0.4129,0.2847,0.5220,0.1101,0.0915,0.0760,0.1808,0.1849,5.1672,0f000001,0*7c4913e5\n\t", "INSPVAXA,USB3,0,48.5,FINESTEERING,2107,281531.950,02000000,471d,15824;INS_ALIGNMENT_COMPLETE,INS_RTKFIXED,37.37125534314,126.72205229379,7.8137,22.3000,-0.0465,0.3065,0.0071,-1.008380878,0.751327706,89.074001876,0.4129,0.2847,0.5220,0.1101,0.0915,0.0760,0.1808,0.1849,5.1672,0f000001,0*42202879\n\t", "INSPVAXA,USB3,0,47.5,FINESTEERING,
